vi "CLD 14 CSV file utility.vi"(8 "Fehler (Eingang)":T1, 11 "CLD 14 - Timer-Enum":T2) -> (0 "Fehler (Ausgang)":T1, 3 "Array":dbl[](array[numeric]))   [LabVIEW 2009]
doc: "Dieses Hilfs-VI liest Daten aus einer *.cvs-Datei aus."
uses:
  <vilib>/Utility/file.llb/Read From Spreadsheet File (string).vi
  CLD 14 CSV file enum.ctl
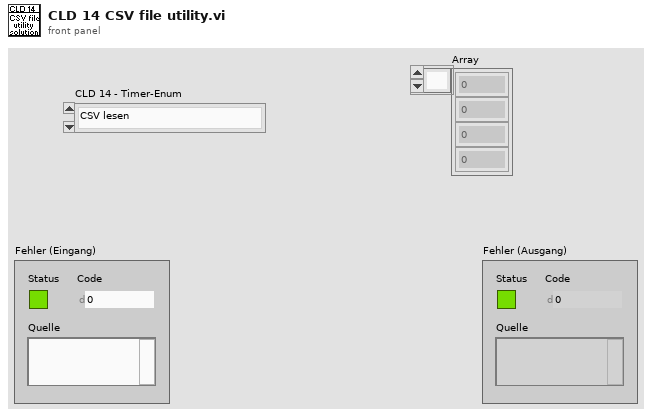
[diagram p1: front panel]
types:
  T1 = cluster{"Status":bool, "Code":i32, "Quelle":string}
  T2 = typedef "CLD 14 CSV file enum.ctl" = enum16{"CSV lesen", "CSV schreiben"}
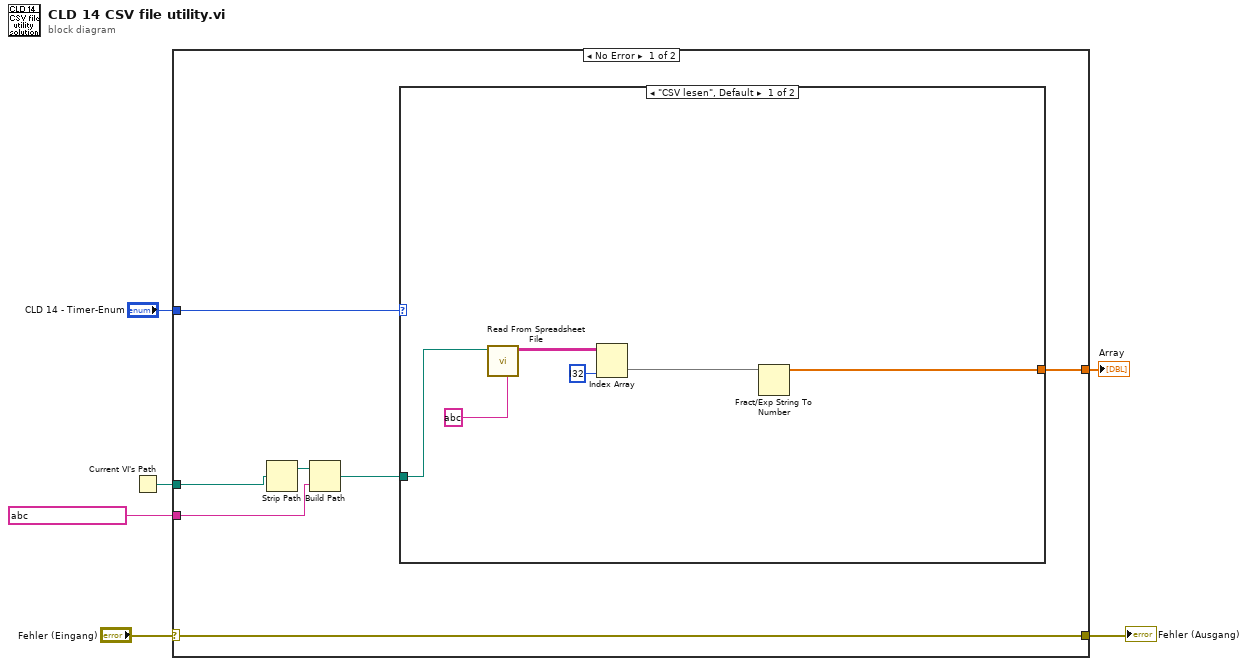
[diagram p0: block diagram]
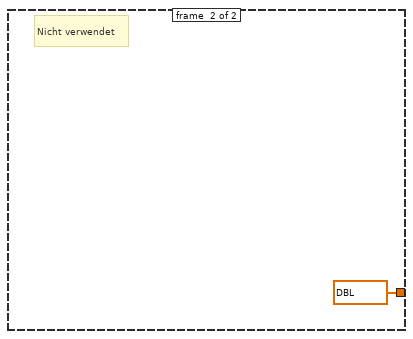
[diagram p2: hidden frame]
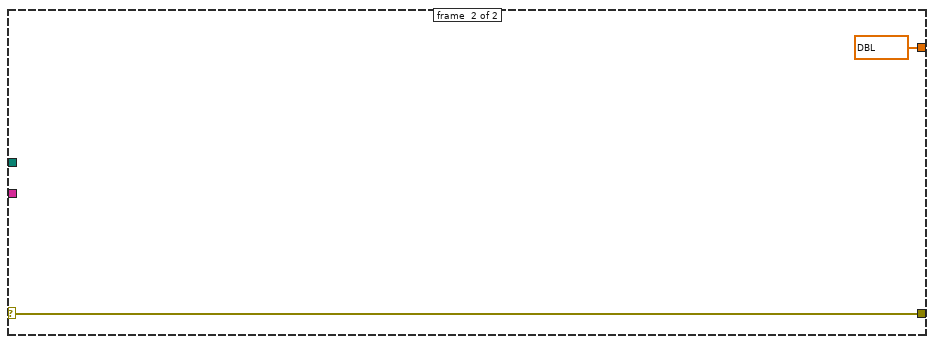
[diagram p3: hidden frame]
diagram:
  n1 = Current VI's Path() -> (path=w5:path)
  n2 = case shown="No Error" "Fehler (Eingang)" {
    selector: "Fehler (Eingang)" -> [w9 w22]
    tunnel: string ? -> [w13 _]
    tunnel: w5 -> [w12 _]
    tunnel: "CLD 14 - Timer-Enum" -> [w10 _]
    tunnel: [w9 w22] -> w2
    tunnel: [w8 dbl[] ?] -> w1
    frame #0 {
      n3 = Strip Path(path=w12) -> (stripped path=w7:path)  [unwired: 1 out]
      n4 = Build Path(base path=w7, name or relative path=w13) -> (appended path=w11:path)
      n5 = case shown="\"CSV lesen\", Default" w10 {
        tunnel: w11 -> [w19 _]
        tunnel: [w14 dbl[] ?] -> w8
        frame #0 {
          n6 = call-poly <vilib>:"Read From Spreadsheet File.vi"("delimiter (\\t)"=string ? ("Trennzeichen (\\t)"), "file path (dialog if empty)"=w19) -> ("all rows"=w17:string[][])  [unwired: 5 in, 4 out]
          n7 = Index Array(array=w17, index (col)=i32 ? ("Deaktivierter Index (Spalte)")) -> (element=w15:string[])  [unwired: 1 in]
          n8 = Fract/Exp String To Number(string=w15) -> (number=w14:dbl[])  [unwired: 3 in, 1 out]
        }
        frame #1 {
          # "Nicht verwendet"
        }
      }
    }
    frame #1 {
    }
  }
  "Fehler (Ausgang)" <- w2
  "Array" <- w1
